vi "build_waveform_cursor.vi"(10 "From [date]":timestamp=timestamp(3629142000 s since 1904-01-01)) -> (2 "Hosszanti irányú gyorsulás":waveform(dbl)(graph) caption="Cursor Waveform")   [LabVIEW 2017]
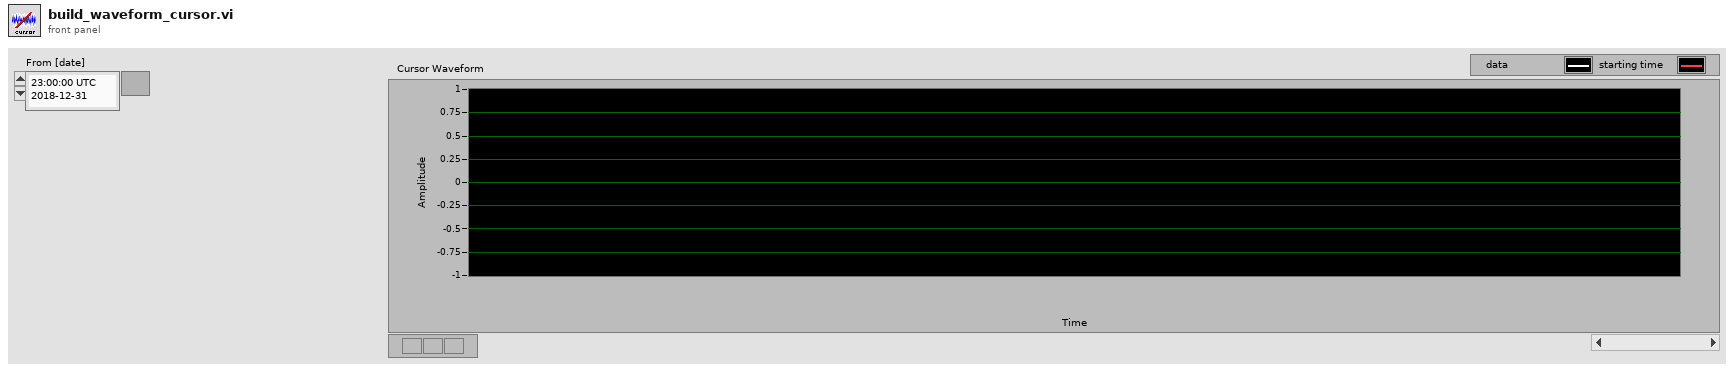
[diagram p1: front panel]
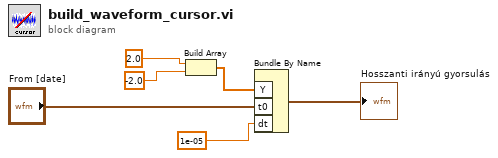
[diagram p0: block diagram]
diagram:
  n1 = Build Array(2.0, -2.0) -> (w5:dbl[])
  n2 = Bundle By Name("Y"=w5, "t0"="From [date]", "dt"=1e-05) -> (→"Hosszanti irányú gyorsulás":waveform(dbl))  [unwired: 1 in]
